vi "Create.vi"(8 "error in (no error)":errorcluster, 9 "Overlay Icon":refnum<class "Icon.lvclass">, 10 "New Name":string="Untitled Project 19", 11 "Destination Directory":path=path "C:/Users/nitest/Documents/LabVIEW Data/Untitled Project 19") -> (0 "error out":errorcluster)   [LabVIEW 2020, in "ADAS_IO_Template_MDO.lvclass"]
uses:
  ADAS_IO_Template_MDO.lvclass
  <vilib>/LabVIEW Icon API/lv_icon/Classes/Icon/Icon.lvclass
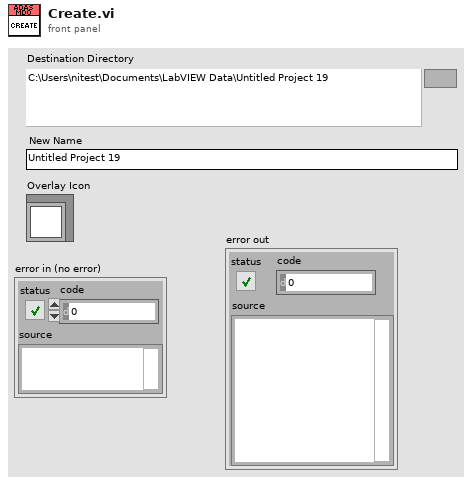
[diagram p1: front panel]
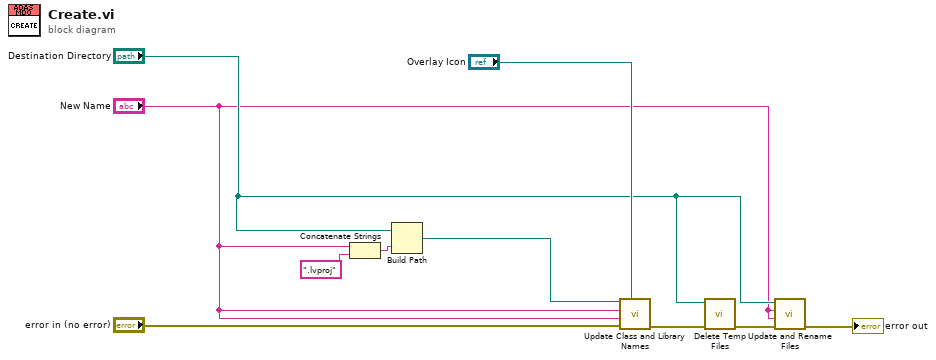
[diagram p0: block diagram]
diagram:
  n1 = Concatenate Strings("New Name", ".lvproj" ("string")) -> (w9:string)
  n2 = Build Path(base path="Destination Directory", name or relative path=w9) -> (appended path=w6:path)
  n3 = call "Update Class and Library Names.vi"("Overlay Icon"="Overlay Icon", "error in (no error)"="error in (no error)", "Type ID"="New Name", "New Name"="New Name", "Project Path"=w6) -> ("error out"=w8:errorcluster)  [unwired: 6 in]
  n4 = call "Delete Temp Files.vi"("error in"=w8, "New PE Folder"="Destination Directory") -> ("error out"=w5:errorcluster)  [unwired: 9 in]
  n5 = call "Update and Rename Files.vi"("error in"=w5, "Type ID"="New Name", "New Name"="New Name", "New PE Folder"="Destination Directory") -> ("error out"=→"error out":errorcluster)  [unwired: 7 in]
